vi "Run Tests - When No Tests Provided - Returns No Results.vi"() -> ()   [LabVIEW 2017, in "LVUnit Test Executor.Tests.lvlib"]
uses:
  LVUnit Test Executor.Tests.lvlib
  LVUnit Test Executor/LVUnit Test Executor.lvclass
  Test Case/Test Case.lvclass
  <vilib>/PNR/Transparent Assertions/Transparent Assertions/Assertions/Assertions.lvlib
  Test Result/Test Result.lvclass
panel:
  out "error out":errorcluster
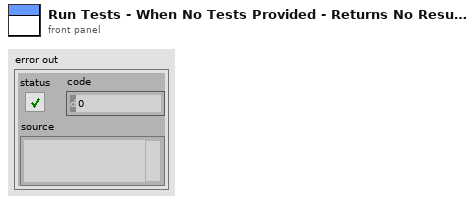
[diagram p1: front panel]
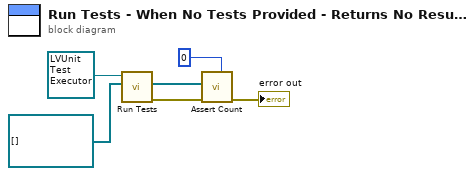
[diagram p0: block diagram]
diagram:
  n1 = call-dynamic "Run Tests.vi"("Test Cases"=refnum<class "Test Case.lvclass">[] [], "LVUnit Test Executor in"=refnum<class "LVUnit Test Executor.lvclass"> refnum ("LVUnit Test Executor")) -> ("error out"=w4:errorcluster, "Test Results"=w3:refnum<class "Test Result.lvclass">[])  [unwired: 7 in, 1 out]
  n2 = call <vilib>:"Assert Count.vi"("Expected"=0, "error in (no error)"=w4, "Haystack"=w3) -> ("error out"=→"error out":errorcluster)  [unwired: 8 in]
